vi "data.vi"(8 "error in (no error)":errorcluster, 11 "VISA resource name":refnum<visa-resource-name>) -> (0 "error out":errorcluster, 2 "Power":dbl, 3 "VISA resource name out":refnum<visa-resource-name>)   [LabVIEW 2013, in "Newport 1830-C.lvlib"]
doc: "AVG?=T, will return average of measurements taken 0.2 s apart for duration of averaging time.\nAVG?=F, will return one measurement.\n\nCurrent Range sets the maximum allowed value. If Power Meter reads during autoranging, will return baloney value, which this screens out and instead returns 0. Default is 10.5W for autoranging. Other ranges only work with ATTN on.\n\nWARNING! Range Query NEVER returns autoranging. If autoranging, set it manually before reading."
uses:
  Newport 1830-C.lvlib
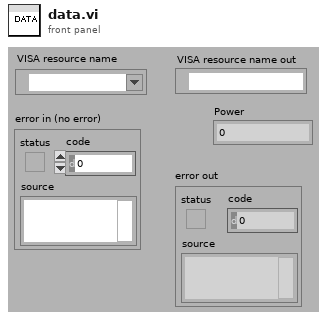
[diagram p1: front panel]
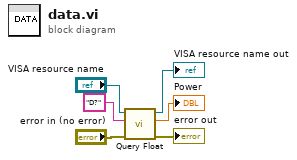
[diagram p0: block diagram]
diagram:
  n1 = call "Query Float.vi"("error in (no error)"="error in (no error)", "write buffer"="D?", "VISA resource name In"="VISA resource name") -> ("error out"=→"error out":errorcluster, "float"=→"Power":dbl, "VISA resource name out"=→"VISA resource name out":refnum<visa-resource-name>)  [unwired: 6 in]
